vi "Write Listener Type.vi"(8 "error in (no error)":errorcluster, 10 "Listener Type":refnum<class "Connection.TCP.lvclass">, 11 "OAuthClient in":refnum<class "OAuthClient.lvclass">) -> (0 "error out":errorcluster, 3 "OAuthClient out":refnum<class "OAuthClient.lvclass">)   [LabVIEW 2013, in "OAuthClient.lvclass"]
uses:
  OAuthClient.lvclass
  <vilib>/LabVIEW Open Source Project/Connection/Connection.TCP/Connection.TCP.lvclass
  OAuthClient.lvclass/OAuthClient.ctl
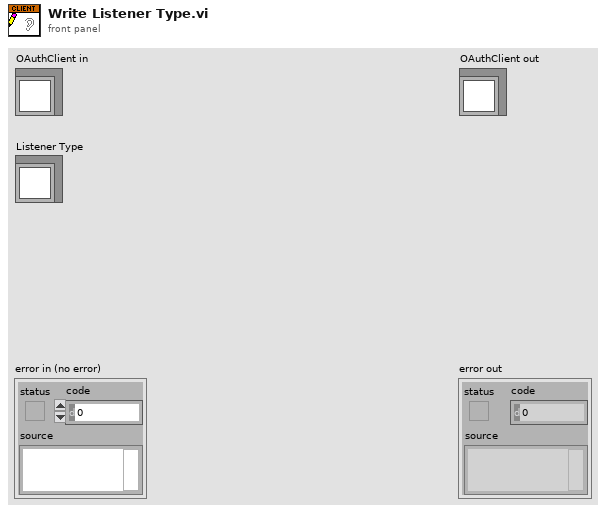
[diagram p1: front panel]
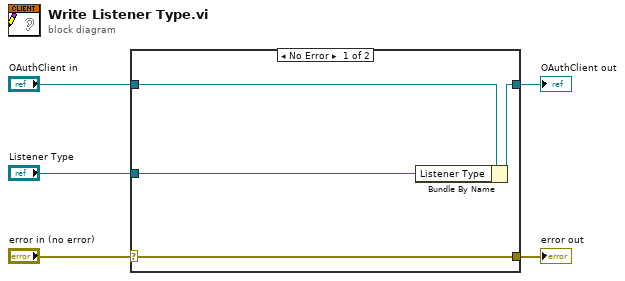
[diagram p0: block diagram]
diagram:
  n1 = case shown="No Error" "error in (no error)" {
    selector: "error in (no error)" -> [w9 w10]
    tunnel: [w9 w10] -> w4
    tunnel: [w7 w11] -> w2
    tunnel: "OAuthClient in" -> [w8 w11]
    tunnel: "Listener Type" -> [w6 _]
    frame No Error {
      n2 = Bundle By Name(cluster=w8, "Listener Type"=w6) -> (w7:refnum<class "OAuthClient.lvclass">)
    }
    frame Error {
    }
  }
  "error out" <- w4
  "OAuthClient out" <- w2
